vi "Mask Neighbors.vi"(11 "Flash Position":cluster{"X":i32, "Y":i32}) -> (3 "Neigbor Mask":i64[][](array[numeric]))   [LabVIEW 2021]
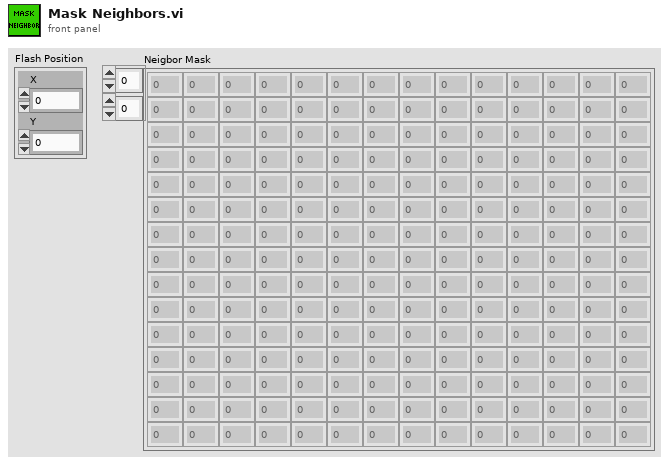
[diagram p1: front panel]
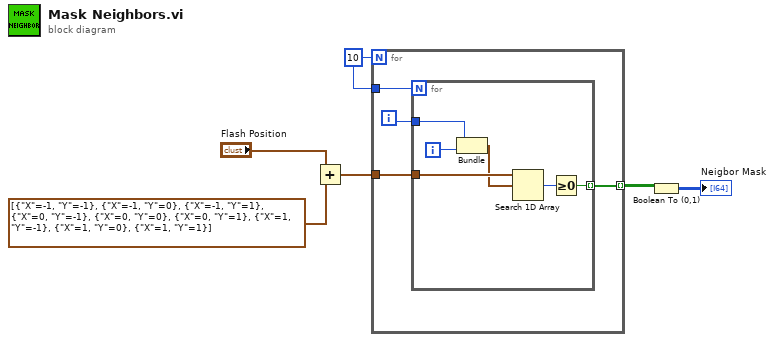
[diagram p0: block diagram]
diagram:
  w1 = 10
  n1 = Add(x="Flash Position", y=cluster{"X":i32, "Y":i32}[] [{"X"=-1, "Y"=-1}, {"X"=-1, "Y"=0}, {"X"=-1, "Y"=1}, {"X"=0, "Y"=-1}, {"X"=0, "Y"=0}, {"X"=0, "Y"=1}, {"X"=1, "Y"=-1}, {"X"=1, "Y"=0}, {"X"=1, "Y"=1}]) -> (x+y=w4:cluster{"X":i32, "Y":i32}[])
  n2 = for {
    N: w1 -> [_]
    tunnel: w4 -> [w10]
    tunnel: [w8] -> w3 mode=indexing
    tunnel: w1 -> [w7]
    i -> [w9]
    n3 = for {
      N: w7 -> [_]
      tunnel: w10 -> [w14]
      tunnel: w9 -> [w15]
      tunnel: [w11] -> w8 mode=indexing
      i -> [w16]
      n4 = Bundle(w15, w16) -> (w13:cluster{i32, i32})  [unwired: 1 in]
      n5 = Search 1D Array(1D array=w14, element=w13) -> (index of element=w12:i32)  [unwired: 1 in]
      n6 = Greater Or Equal To 0?(x=w12) -> (x >= 0?=w11:bool)
    }
  }
  n7 = Boolean To (0,1)(Boolean=w3) -> (0, 1=→"Neigbor Mask":i16[][])
